vi "Read FocusObj.vi"(8 "error in (no error)":errorcluster, 11 "ControlKeyUpMsg in":refnum<class "ControlKeyUpMsg.lvclass">) -> (0 "error out":errorcluster, 2 "FocusObj":refnum<vi>, 3 "ControlKeyUpMsg out":refnum<class "ControlKeyUpMsg.lvclass">)   [LabVIEW 2020, in "MVA Framework.lvlib" / "ActorEvents.lvlib" / "ControlKeyUpMsg.lvclass"]
uses:
  ControlKeyUpMsg.lvclass
  ControlKeyUpMsg.lvclass/ControlKeyUpMsg.ctl
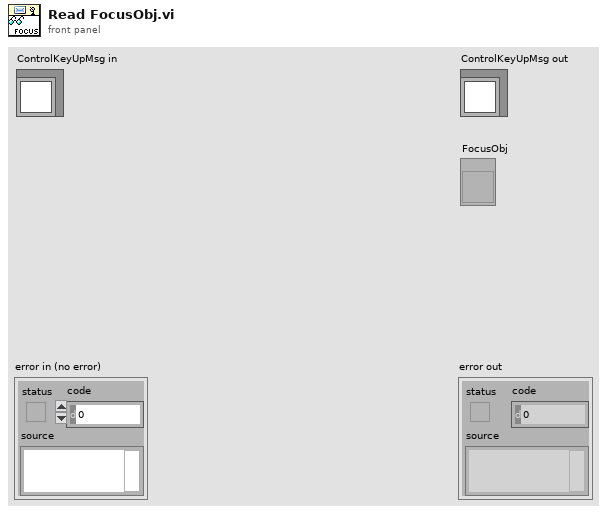
[diagram p1: front panel]
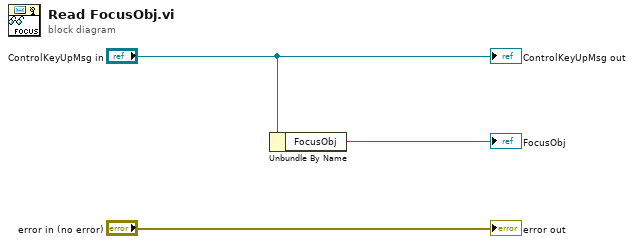
[diagram p0: block diagram]
diagram:
  n1 = Unbundle By Name("ControlKeyUpMsg in") -> ("FocusObj"=→"FocusObj":refnum<vi>)
  "error out" <- "error in (no error)"
  "ControlKeyUpMsg out" <- "ControlKeyUpMsg in"
